vi "Realarmctrl.vi"() -> ()   [LabVIEW 2024]
panel:
  out "resulting string":string
  in  "geometry?":bool=TRUE
  in  "dx":dbl=10.0
  in  "dy":dbl
  in  "bias":dbl
  in  "v":dbl=100.0
  in  "L 1":dbl(slide)=30.0 scale=0.0..200.0
  in  "L 2":dbl(slide)=30.0 scale=0.0..200.0
  out "2D Picture":picture
  out "output cluster":cluster{"L 1":dbl, "L 2":dbl, "q":dbl[]}
  out "vq":dbl[](array[numeric]) format="%.2f"
  in  "Timeout (ms)":u32=1000
  in  "VISA Refnum in":refnum<visa-resource-name>
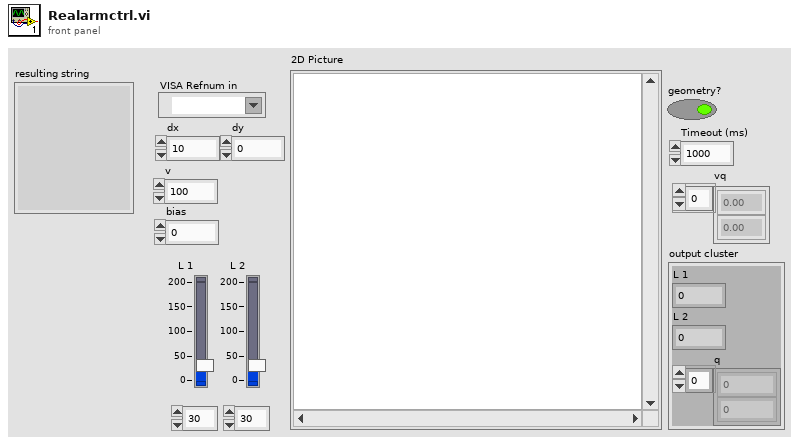
[diagram p1: front panel]
types:
  T1 = cluster{"Width":u16, "Style":enum32{"Solid", "Dash", "Dot", "DashDot", "DashDotDot"}}
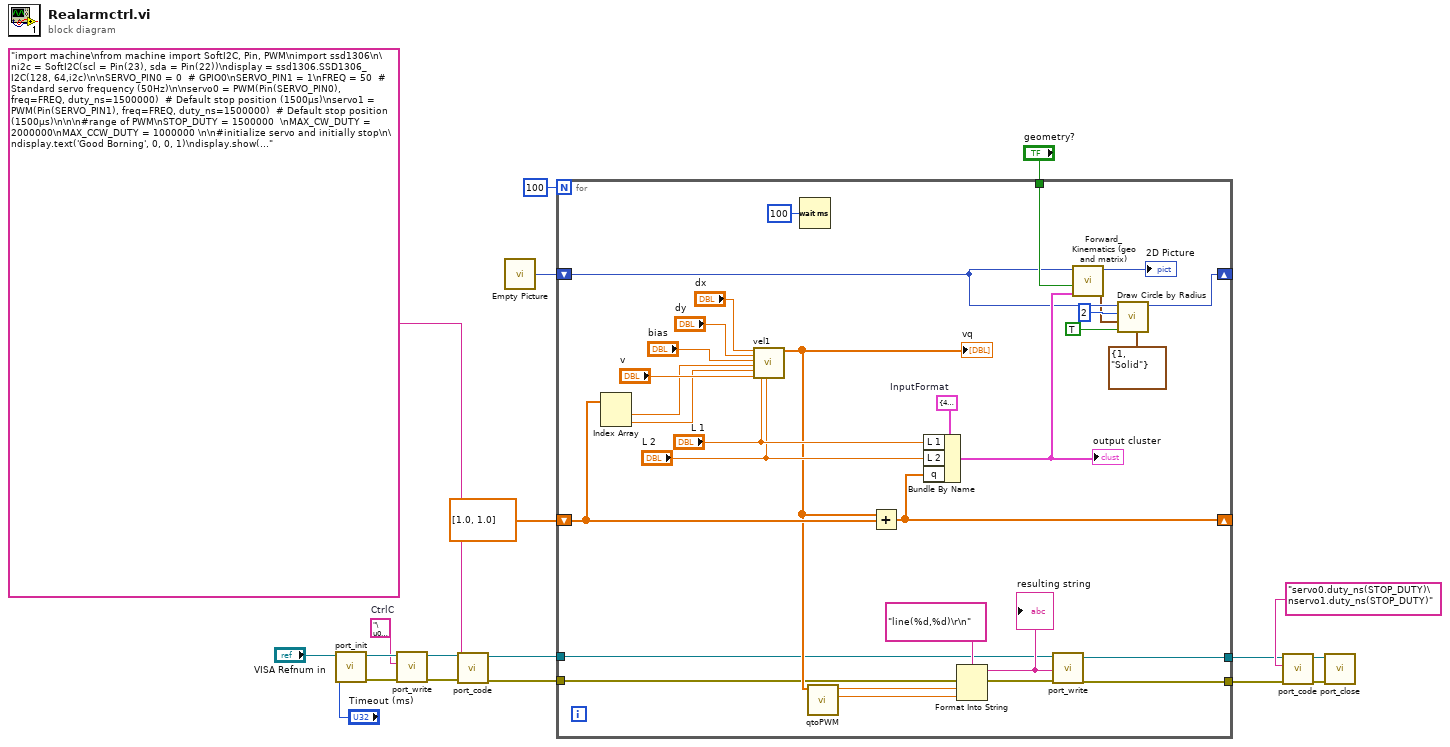
[diagram p0: block diagram]
diagram:
  w13 = "\u0003"  # CtrlC
  n1 = call <userlib>:"port_init.vi"("Timeout (ms)"="Timeout (ms)", "VISA Refnum in"="VISA Refnum in") -> ("error out"=w16:errorcluster, "VISA Refnum out"=w17:refnum<visa-resource-name>)  [unwired: 8 in]
  n2 = call <userlib>:"port_write.vi"("error in (no error)"=w16, "write buffer"=w13, "VISA Refnum in"=w17) -> ("error out"=w14:errorcluster, "VISA Refnum out"=w15:refnum<visa-resource-name>)  [unwired: 7 in]
  n3 = call <userlib>:"port_code.vi"("error in (no error)"=w14, "Code to run"="import machine\nfrom machine import SoftI2C, Pin, PWM\nimport ssd1306\n\ni2c = SoftI2C(scl = Pin(23), sda = Pin(22))\ndisplay = ssd1306.SSD1306_I2C(128, 64,i2c)\n\nSERVO_PIN0 = 0  # GPIO0\nSERVO_PIN1 = 1\nFREQ = 50  # Standard servo frequency (50Hz)\n\nservo0 = PWM(Pin(SERVO_PIN0), freq=FREQ, duty_ns=1500000)  # Default stop position (1500μs)\nservo1 = PWM(Pin(SERVO_PIN1), freq=FREQ, duty_ns=1500000)  # Default stop position (1500μs)\n\n\n#range of PWM\nSTOP_DUTY = 1500000  \nMAX_CW_DUTY = 2000000\nMAX_CCW_DUTY = 1000000 \n\n#initialize servo and initially stop\n\ndisplay.text('Good Borning', 0, 0, 1)\ndisplay.show()\n\nservo0.duty_ns(STOP_DUTY)\nservo1.duty_ns(STOP_DUTY)\n\ndef line(a0, a1):\n    display.fill(0)\n    display.text(\"a0: \" + str(a0), 0, 0, 1)\n    display.text(\"a1: \" + str(a1), 0, 10, 1)\n    display.text(\"I'm good\" , 10, 20, 1)\n    display.show()\n    servo0.duty_ns(a0*1000)\n    servo1.duty_ns(a1*1000)\n\n\n", "VISA Refnum in"=w15) -> ("error out"=w6:errorcluster, "VISA Refnum out"=w7:refnum<visa-resource-name>)  [unwired: 7 in]
  n4 = call "Empty Picture"() -> ("empty picture"=w8:picture)
  n5 = for {
    N: 100 -> [_]
    tunnel: "geometry?" -> [w43]
    shift-right: [w36] -> _
    shift-left: dbl[] [1.0, 1.0] -> [w39]
    shift-right: [w34] -> _
    shift-left: w8 -> [w32]
    tunnel: w7 -> [w25]
    tunnel: w6 -> [w24]
    tunnel: [w23] -> w2
    tunnel: [w22] -> w1
    w47 = cluster{"L 1":dbl, "L 2":dbl, "q":dbl[]} {"L 1"=40.0, "L 2"=35.0, "q"=[180.0, 60.0]}  # InputFormat
    n6 = Index Array(array=w39) -> (element #1=w38:dbl, element #2=w37:dbl)  [unwired: 2 in]
    n7 = call "vel1.vi"("dx"="dx", "dy"="dy", "bias"="bias", "Angle1"=w38, "Angle 2"=w37, "v"="v", "L 1"="L 1", "L 2"="L 2") -> ("vq"=w29:dbl[])  [unwired: 10 in, 1 out]
    "vq" <- w29
    n8 = Wait (ms)(milliseconds to wait=u32 100) -> ()  [unwired: 1 out]
    n9 = call "qtoPWM.vi"("vq"=w29) -> ("Numeric 2"=w21:dbl, "Numeric"=w20:dbl)  [unwired: 9 in]
    n10 = Add(x=w29, y=w39) -> (x+y=w36:dbl[])
    n11 = Bundle By Name(cluster=w47, "L 1"="L 1", "L 2"="L 2", "q"=w36) -> (w44:cluster{"L 1":dbl, "L 2":dbl, "q":dbl[]})
    "output cluster" <- w44
    n12 = Format Into String(format string="line(%d,%d)\r\n", error in=w24, w20, w21) -> (resulting string=w28:string, error out=w27:errorcluster)  [unwired: 1 in]
    "resulting string" <- w28
    n13 = call <userlib>:"port_write.vi"("error in (no error)"=w27, "write buffer"=w28, "VISA Refnum in"=w25) -> ("error out"=w22:errorcluster, "VISA Refnum out"=w23:refnum<visa-resource-name>)  [unwired: 7 in]
    n14 = call <userlib>:"Forward_Kinematics (geo and matrix).vi"("geometry"=w44, "geometry?"=w43, "picture in"=w32) -> ("end (2D)"=w31:cluster{"x":dbl, "y":dbl}, "2D Picture"=→"2D Picture":picture)  [unwired: 6 in, 1 out]
    n15 = call <vilib>:"Draw Circle by Radius.vi"("pen"=T1 {"Width"=1, "Style"=enum."Solid"}, "fill?(F)"=TRUE, "pixel center"=w31, "radius"=i16 2, "picture"=w32) -> ("new picture"=w34:picture)  [unwired: 6 in]
  }
  n16 = call <userlib>:"port_code.vi"("error in (no error)"=w1, "Code to run"="servo0.duty_ns(STOP_DUTY)\nservo1.duty_ns(STOP_DUTY)", "VISA Refnum in"=w2) -> ("error out"=w3:errorcluster, "VISA Refnum out"=w4:refnum<visa-resource-name>)  [unwired: 7 in]
  n17 = call <userlib>:"port_close.vi"("error in (no error)"=w3, "VISA Refnum in"=w4) -> ()  [unwired: 10 in]
